vi "Example-SPI.vi"() -> ()   [LabVIEW 2018]
panel:
  out "数值":i32
  out "波形图":u8[](graph)
  out "SerialNumber":string
  out "rxcount out":i32
  out "rgRX":u8[](array[numeric])
  in  "Tx data":u8[](array[numeric])
  in  "RX IO(0~15)":i32=1
  in  "TX IO(0~15)":i32
  in  "Frequency(Hz)":i32(ring)=9600 items=["110"=110, "150"=150, "300"=300, "600"=600, "1200"=1200, "2400"=2400, "4800"=4800, "9600"=9600, "14400"=14400, "19200"=19200, "28800"=28800, "38400"=38400, "56000"=56000, "57600"=57600, "115200"=115200, "128000"=128000, "153600"=153600, "230400"=230400, "256000"=256000, "406800"=406800, "921600"=921600]
  out "returns":i32[](array[numeric])
  out "error out":errorcluster caption="错误输出"
  in  "error in (no error)":errorcluster caption="错误输入（无错误）"
  out "ftHandle out":u64=363562184
  in  "设备索引":i32
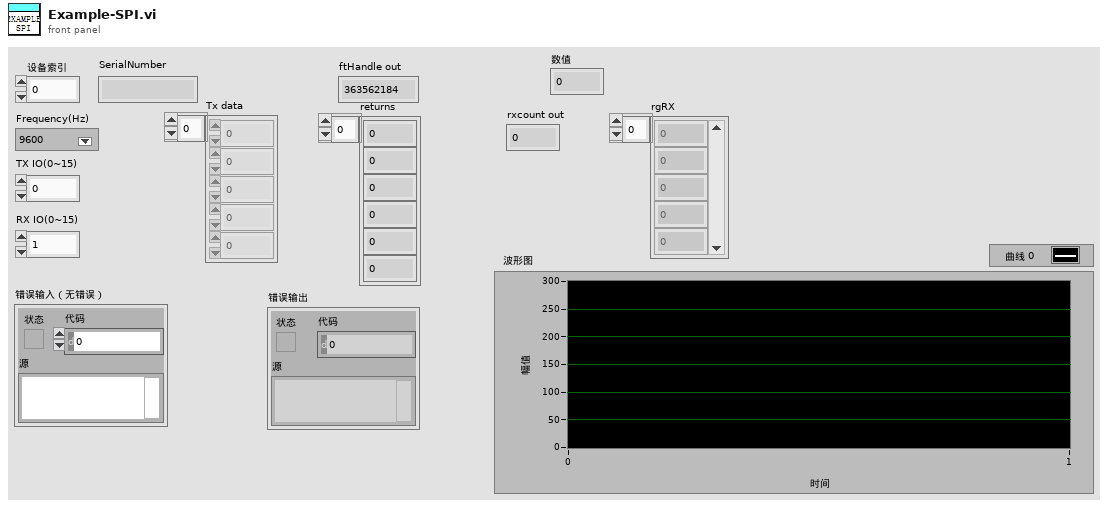
[diagram p1: front panel]
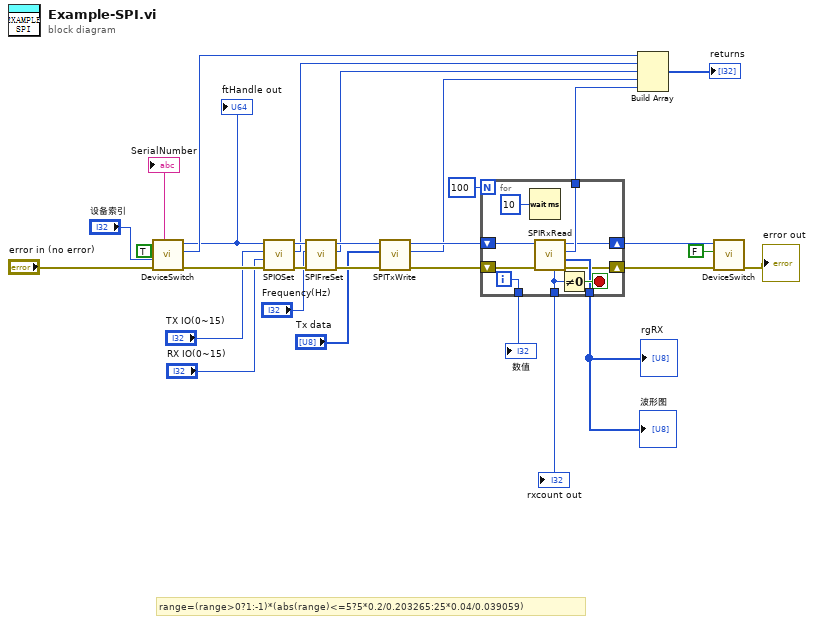
[diagram p0: block diagram]
diagram:
  # "range=(range>0?1:-1)*(abs(range)<=5?5*0.2/0.203265:25*0.04/0.039059)"
  n1 = call "DeviceSwitch.vi"("error in (no error)"="error in (no error)", "Device Index"="设备索引", "Open"=TRUE) -> ("error out"=w15:errorcluster, "function return"=w26:i32, "handle out"=w8:u64, "SerialNumber"=→"SerialNumber":string)  [unwired: 4 in, 1 out]
  "ftHandle out" <- w8
  n2 = call "SPIOSet.vi"("error in (no error)"=w15, "Clock IO(0~15)"="RX IO(0~15)", "CSIO(0~15)"="TX IO(0~15)", "handle"=w8) -> ("error out"=w14:errorcluster, "function return"=w4:i32, "handle out"=w9:u64)  [unwired: 5 in]
  n3 = call "SPIFreSet.vi"("error in (no error)"=w14, "Frequency(Hz)"="Frequency(Hz)", "handle"=w9) -> ("error out"=w13:errorcluster, "function return"=w3:i32, "handle out"=w10:u64)  [unwired: 6 in]
  n4 = call "SPITxWrite.vi"("error in (no error)"=w13, "data"="Tx data", "handle"=w10) -> ("error out"=w12:errorcluster, "function return"=w2:i32, "handle out"=w11:u64)  [unwired: 6 in]
  n5 = for {
    N: 100 -> [_]
    tunnel: [w35] -> w21
    tunnel: [w33] -> w17
    tunnel: [w31] -> w19
    shift-right: [w32] -> w23
    shift-left: w12 -> [w37]
    shift-right: [w34] -> w22
    shift-left: w11 -> [w36]
    tunnel: [w38] -> w16
    i -> [w38]
    stop <- w40 stop-if-true
    n6 = Wait (ms)(milliseconds to wait=u32 10 ("等待时间（毫秒）")) -> ()  [unwired: 1 out]
    n7 = call "SPIRxRead.vi"("error in (no error)"=w37, "handle"=w36) -> ("error out"=w32:errorcluster, "rgRX"=w33:u8[], "function return"=w35:i32, "handle out"=w34:u64, "rxcount out"=w31:i32)  [unwired: 5 in]
    n8 = Not Equal To 0?(x=w31) -> (x != 0?=w40:bool)
  }
  "rgRX" <- w17
  "rxcount out" <- w19
  "波形图" <- w17
  "数值" <- w16
  n9 = Build Array(w26, w4, w3, w2, w21) -> (→"returns":i32[])
  n10 = call "DeviceSwitch.vi"("error in (no error)"=w23, "Open"=FALSE, "handle"=w22) -> ("error out"=→"error out":errorcluster)  [unwired: 4 in, 4 out]
